vi "Memory.Pointer.Parameter Check.Subset.vi"(7 "source vi name":string, 8 "error in (no error)":errorcluster, 9 "offset (0)":u64 format="%08x bytes", 10 "length":u64 format="%08x bytes", 11 "Pointer in":refnum<class "Memory.Pointer.lvclass">) -> (0 "error out":errorcluster, 1 "offset out":u64 format="%08x bytes", 2 "length":u64 format="%08x bytes", 3 "Pointer out":refnum<class "Memory.Pointer.lvclass">)   [LabVIEW 2016, in "Memory Manager.lvlib" / "Memory.Pointer.lvclass"]
uses:
  Memory.Pointer.lvclass
  Memory.Pointer.lvclass/Memory.Pointer.ctl
  Memory.Pointer.Errors.Out of Bounds.vi
  Submodules/SEH/Source/VIs/Static Error Handling.Source Buffer.Write.String.vi
  Memory.Pointer.Errors.Write Pointer Size.vi
  Memory.Pointer.Errors.Create Error.vi
  Submodules/SEH/Source/VIs/Static Error Handling.Source Buffer.Write.Numeric.Scalar.Base10.vi
  Submodules/SEH/Source/VIs/Static Error Handling.Source Buffer.Write.Numeric.Scalar.Base10 (U64).vi
  Submodules/SEH/Source/VIs/Static Error Handling.Error Cluster Constant.vi
  Submodules/SEH/Source/VIs/Static Error Handling.Error Cluster Constant (256B).vi
  Submodules/SEH/Source/VIs/Static Error Handling.Parameters.Status.Set.vi
  Submodules/SEH/Source/VIs/Static Error Handling.Parameters.Code.Set.vi
  Submodules/SEH/Source/VIs/Static Error Handling.Parameters.VI Source.Set.vi
  Constants/Memory.Constants.vi
  Constants/Memory.Constants.Library Name.vi
  Memory.Pointer.Errors.Get Info.vi
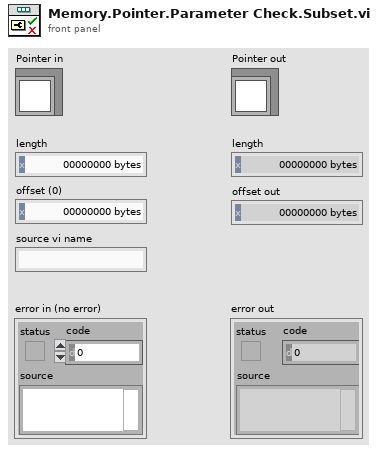
[diagram p1: front panel]
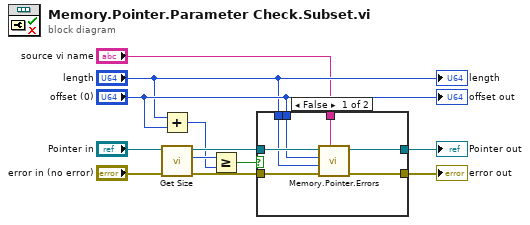
[diagram p0: block diagram]
diagram:
  n1 = Add(x="length", y="offset (0)") -> (x+y=w1:u64)
  n2 = call "Get Size.vi"("error in (no error)"="error in (no error)", "Pointer in"="Pointer in") -> ("error out"=w7:errorcluster, "size"=w10:u64, "Pointer out"=w3:refnum<class "Memory.Pointer.lvclass">)  [unwired: 7 in]
  n3 = Greater Or Equal?(x=w10, y=w1) -> (x >= y?=w6:bool)
  n4 = case shown="False" w6 {
    tunnel: w3 -> [w19 w20]
    tunnel: w7 -> [w17 w21]
    tunnel: [w16 w21] -> w12
    tunnel: [w18 w20] -> w11
    tunnel: "offset (0)" -> [w15 _]
    tunnel: "length" -> [w14 _]
    tunnel: "source vi name" -> [w13 _]
    frame False {
      n5 = call-poly "Memory.Pointer.Errors.vi"("source vi name"=w13, "error in (no error)"=w17, "length"=w14, "offset"=w15, "pointer in"=w19) -> ("error out"=w16:errorcluster, "pointer out"=w18:refnum<class "Memory.Pointer.lvclass">)  [unwired: 5 in]
    }
    frame True {
    }
  }
  "error out" <- w12
  "Pointer out" <- w11
  "offset out" <- "offset (0)"
  "length" <- "length"
